vi "PC_Shot_Power.vi"(5 "Bounce T/F?":bool, 7 "Puck Selection":enum32{"PTFE", "Nylon"}(radio), 8 "Error In":errorcluster, 11 "PC Data":T1) -> (0 "Error Out":errorcluster, 2 "Kicker angle":dbl, 3 "Power %":dbl)   [LabVIEW 2017]
uses:
  pc_data.ctl
  <vilib>/vision/Image Controls.llb/IMAQ Image.ctl
  <vilib>/Utility/file.llb/Read Delimited Spreadsheet (DBL).vi
panel:
  in  "FF Bounce":dbl=0.66
  in  "FF Straight":dbl=1.68 format="%#_13g"
  out "Goal Y Bounce":dbl
  in  "Kicker Res":dbl=0.5
  out "Goal Y Straight":dbl
  in  "Friction PTFE":dbl=0.4
  in  "Puck Mass PTFE":dbl=0.0069
  in  "Friction Nylon":dbl=0.31
  in  "Puck Mass Nylon":dbl=0.0037
  out "Wall X Bounce":dbl
  out "Pot Position":dbl
  in  "Pendulum length":dbl=0.069
  in  "Pendulum mass":dbl=0.096
  out "Required E":dbl
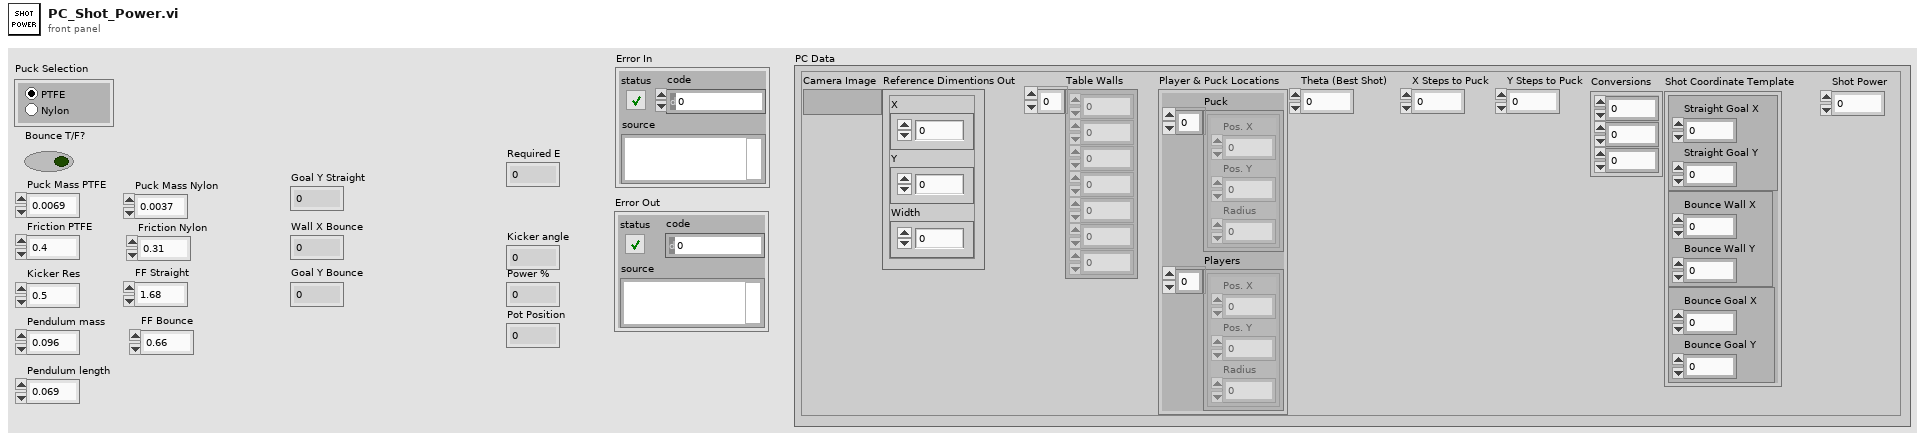
[diagram p1: front panel]
types:
  T1 = typedef "pc_data.ctl" = cluster{"Camera Image":T2, "Reference Dimentions Out":cluster{"X":dbl, "Y":dbl, "Width":dbl}, "Table Walls":sgl[], "Player & Puck Locations":cluster{"Puck":cluster{"Pos. X":i32, "Pos. Y":i32, "Radius":i32}[], "Players":cluster{"Pos. X":i32, "Pos. Y":i32, "Radius":i32}[]}, "Theta (Best Shot)":dbl, "X Steps to Puck":dbl, "Y Steps to Puck":dbl, "Conversions":cluster{dbl, dbl, dbl}, "Shot Coordinate Template":cluster{cluster{"Straight Goal X":sgl, "Straight Goal Y":dbl}, cluster{"Bounce Wall X":dbl, "Bounce Wall Y":sgl}, cluster{"Bounce Goal X":sgl, "Bounce Goal Y":dbl}}, "Shot Power":dbl}
  T2 = typedef "IMAQ Image.ctl" = refnum<image>
  T3 = cluster{"Pos. X":i32, "Pos. Y":i32, "Radius":i32}[]
  T4 = cluster{cluster{"Straight Goal X":sgl, "Straight Goal Y":dbl}, cluster{"Bounce Wall X":dbl, "Bounce Wall Y":sgl}, cluster{"Bounce Goal X":sgl, "Bounce Goal Y":dbl}}
  T5 = cluster{"Straight Goal X":sgl, "Straight Goal Y":dbl}
  T6 = cluster{"Bounce Wall X":dbl, "Bounce Wall Y":sgl}
  T7 = cluster{"Bounce Goal X":sgl, "Bounce Goal Y":dbl}
  T8 = cluster{"Pos. X":i32, "Pos. Y":i32, "Radius":i32}
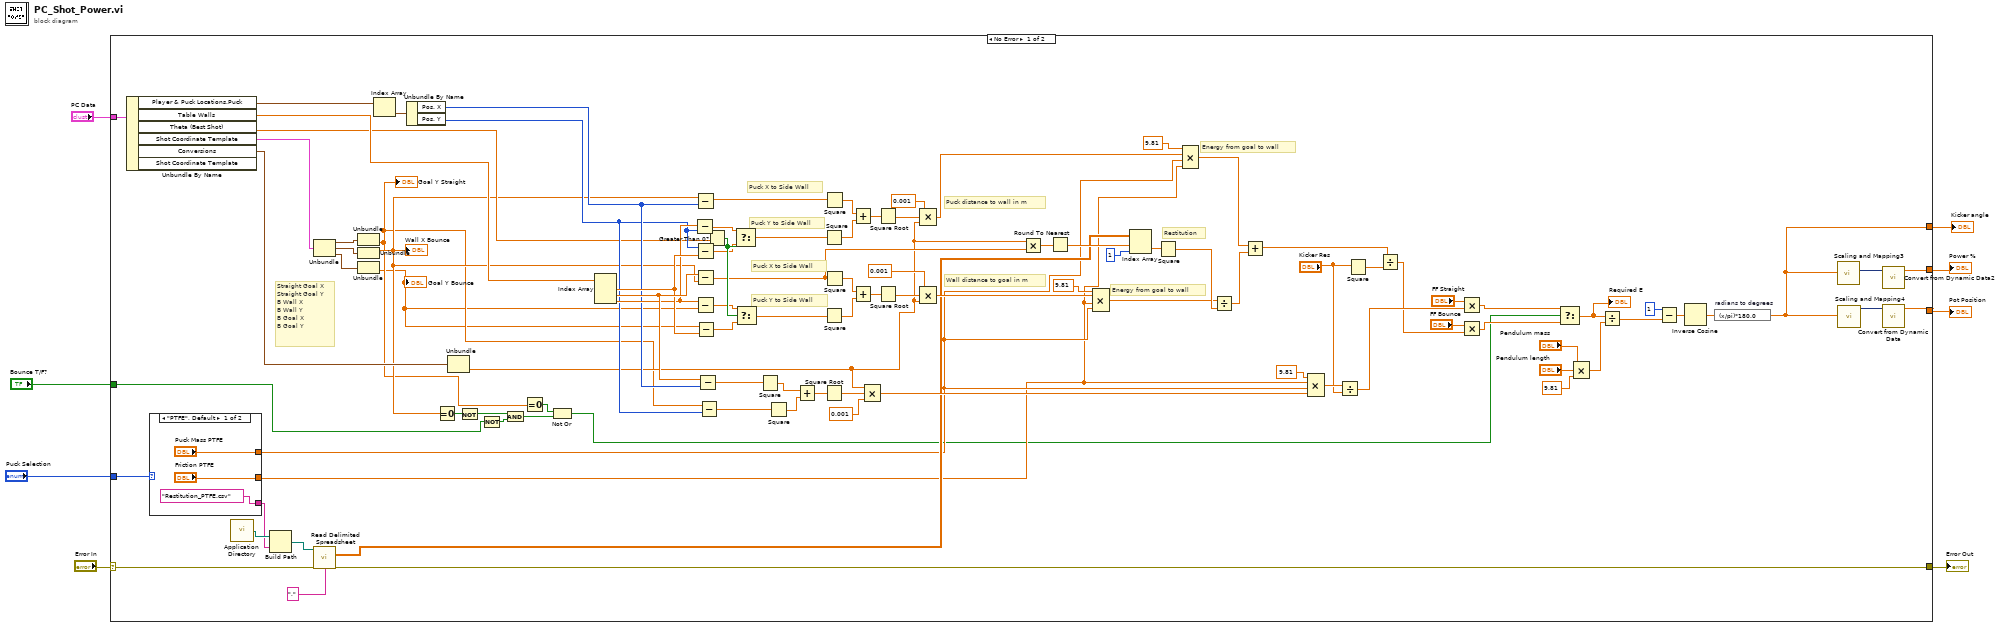
[diagram p0: block diagram]
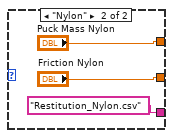
[diagram p2: hidden frame]
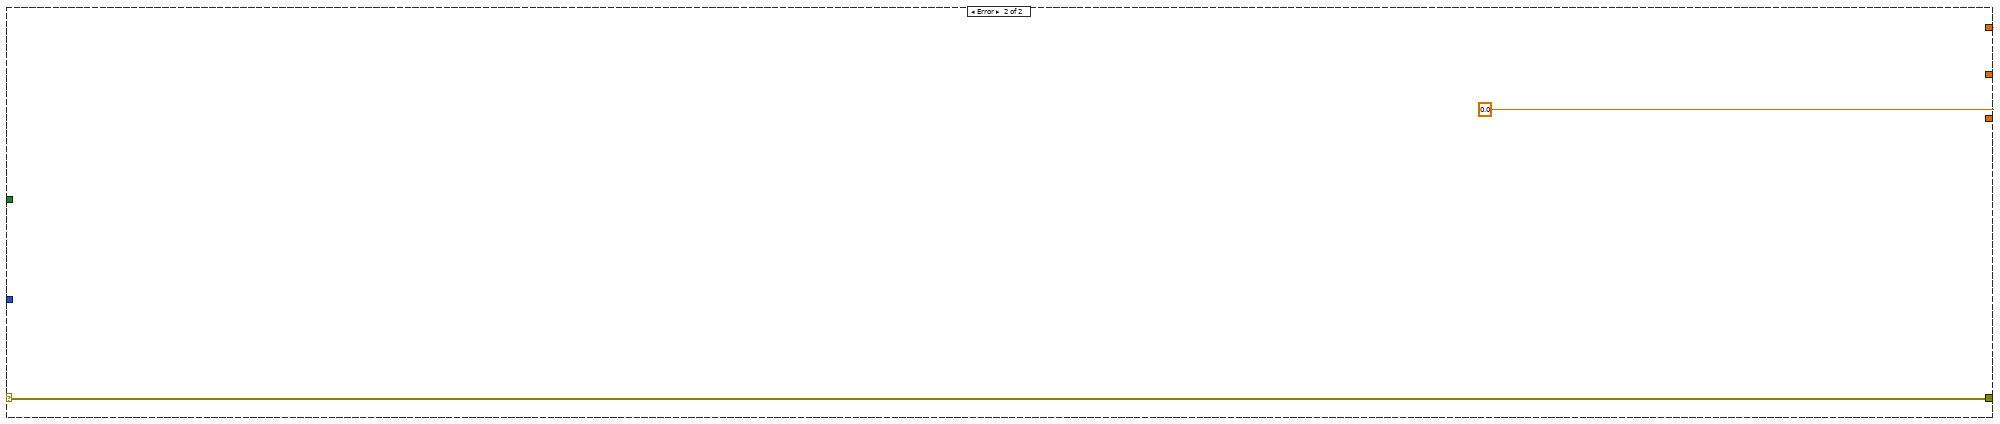
[diagram p3: hidden frame]
diagram:
  n1 = case shown="No Error" "Error In" {
    selector: "Error In" -> [w107 w116]
    tunnel: [w106 w116] -> w7
    tunnel: "Puck Selection" -> [w105 _]
    tunnel: "PC Data" -> [w102 _]
    tunnel: [w24 0.0] -> w4
    tunnel: [w25 _] -> w3
    tunnel: [w22 _] -> w2
    tunnel: "Bounce T/F?" -> [w13 _]
    frame No Error {
      # "Energy from goal to wall"
      # "Restitution"
      # "Energy from goal to wall"
      # "Puck X to Side Wall"
      # "Puck Y to Side Wall"
      # "Wall distance to goal in m"
      # "Puck distance to wall in m"
      # "Puck Y to Side Wall"
      # "Puck X to Side Wall"
      # "Straight Goal X\nStraight Goal Y\nB Wall X\nB Wall Y\nB Goal X\nB Goal Y"
      n2 = Unbundle By Name(w102) -> ("Player & Puck Locations.Puck"=w104:T3, "Table Walls"=w37:sgl[], "Theta (Best Shot)"=w34:dbl, "Shot Coordinate Template"=w98:T4, "Conversions"=w94:cluster{dbl, dbl, dbl})  [unwired: 1 out]
      n3 = case shown="\"PTFE\", Default" w105 {
        tunnel: ["Puck Mass PTFE" "Puck Mass Nylon"] -> w31
        tunnel: ["Friction PTFE" "Friction Nylon"] -> w30
        tunnel: ["Restitution_PTFE.csv" "Restitution_Nylon.csv"] -> w99
        frame "PTFE", Default {
        }
        frame "Nylon" {
        }
      }
      n4 = call <vilib>:"Application Directory.vi"() -> ("Application Directory"=w100:path)
      n5 = Build Path(base path=w100, name or relative path=w99) -> (appended path=w101:path)
      n6 = Unbundle(w98) -> (w97:T5, w96:T6, w95:T7)
      n7 = call-poly <vilib>:"Read Delimited Spreadsheet.vi"("file path (dialog if empty)"=w101, "error in (no error)"=w107, "delimiter (\\t)"="," ("delimiter (\\t)")) -> ("all rows"=w32:dbl[][], "error out"=w106:errorcluster)  [unwired: 7 in, 4 out]
      n8 = Unbundle(w97) -> ("Straight Goal Y"=w10:dbl)  [unwired: 1 out]
      "Goal Y Straight" <- w10
      n9 = Unbundle(w96) -> ("Bounce Wall X"=w11:dbl)  [unwired: 1 out]
      "Wall X Bounce" <- w11
      n10 = Unbundle(w95) -> ("Bounce Goal Y"=w9:dbl)  [unwired: 1 out]
      "Goal Y Bounce" <- w9
      n11 = Index Array(array=w104) -> (element=w103:T8)  [unwired: 1 in]
      n12 = Unbundle By Name(w103) -> ("Pos. X"=w36:i32, "Pos. Y"=w35:i32)
      n13 = Equal To 0?(x=w11) -> (x = 0?=w17:bool)
      n14 = Unbundle(w94) -> (w33:dbl)  [unwired: 2 out]
      n15 = Not(x=w17) -> (.not. x?=w16:bool)
      n16 = Not(x=w13) -> (.not. x?=w15:bool)
      n17 = And(x=w16, y=w15) -> (x .and. y?=w18:bool)
      n18 = Equal To 0?(x=w10) -> (x = 0?=w12:bool)
      n19 = Not Or(1:w18, 2:w12) -> (0:w14:bool)
      n20 = Index Array(array=w37) -> (element #1=w62:sgl, element #2=w84:sgl, element #3=w61:sgl)  [unwired: 3 in]
      n21 = Subtract(x=w61, y=w35) -> (x-y=w47:sgl)
      n22 = Subtract(x=w11, y=w36) -> (x-y=w50:dbl)
      n23 = Subtract(x=w35, y=w62) -> (x-y=w48:sgl)
      n24 = Subtract(x=w84, y=w11) -> (x-y=w65:dbl)
      n25 = Subtract(x=w61, y=w9) -> (x-y=w60:dbl)
      n26 = Subtract(x=w9, y=w62) -> (x-y=w59:dbl)
      n27 = Subtract(x=w84, y=w36) -> (x-y=w81:sgl)
      n28 = Subtract(x=w10, y=w35) -> (x-y=w80:dbl)
      n29 = Greater Than 0?(x=w34) -> (x > 0?=w85:bool)
      n30 = Select(t=w47, s=w85, f=w48) -> (s? t:f=w49:sgl)
      n31 = Select(t=w60, s=w85, f=w59) -> (s? t:f=w63:dbl)
      n32 = Square(x=w81) -> (x^2=w78:sgl)
      n33 = Square(x=w80) -> (x^2=w79:dbl)
      n34 = Add(x=w78, y=w79) -> (x+y=w77:dbl)
      n35 = Square(x=w49) -> (x^2=w52:sgl)
      n36 = Square(x=w63) -> (x^2=w57:dbl)
      n37 = Square Root(x=w77) -> (sqrt(x)=w76:dbl)
      n38 = Square(x=w50) -> (x^2=w51:dbl)
      n39 = Square(x=w65) -> (x^2=w58:dbl)
      n40 = Add(x=w51, y=w52) -> (x+y=w53:dbl)
      n41 = Add(x=w58, y=w57) -> (x+y=w56:dbl)
      n42 = Compound Arithmetic op=MULTIPLY(w33, w76, 0.001 ("value")) -> (w82:dbl)
      n43 = Square Root(x=w53) -> (sqrt(x)=w54:dbl)
      n44 = Square Root(x=w56) -> (sqrt(x)=w55:dbl)
      n45 = Compound Arithmetic op=MULTIPLY(0.001 ("value"), w54, w33) -> (w70:dbl)
      n46 = Compound Arithmetic op=MULTIPLY(0.001 ("value"), w55, w33) -> (w64:dbl)
      n47 = Multiply(x=w33, y=w65) -> (x*y=w66:dbl)
      n48 = Round To Nearest(number=w66) -> (nearest integer value=w67:dbl)
      n49 = Compound Arithmetic op=MULTIPLY(9.81 ("value"), w64, w30, w31) -> (w69:dbl)
      n50 = Index Array(array=w32, index (row)=w67, index (col)=1 ("disabled index (col)")) -> (element=w68:dbl)
      n51 = Square(x=w68) -> (x^2=w73:dbl)
      n52 = Compound Arithmetic op=MULTIPLY(9.81 ("value"), w70, w31, w30) -> (w72:dbl)
      n53 = Divide(x=w69, y=w73) -> (x/y=w71:dbl)
      n54 = Add(x=w72, y=w71) -> (x+y=w75:dbl)
      n55 = Compound Arithmetic op=MULTIPLY(9.81 ("value"), w30, w31, w82) -> (w83:dbl)
      n56 = Divide(x=w83, y="Kicker Res") -> (x/y=w90:dbl)
      n57 = Square(x="Kicker Res") -> (x^2=w74:dbl)
      n58 = Divide(x=w75, y=w74) -> (x/y=w21:dbl)
      n59 = Multiply(x="FF Straight", y=w90) -> (x*y=w92:dbl)
      n60 = Multiply(x="FF Bounce", y=w21) -> (x*y=w20:dbl)
      n61 = Select(t=w92, s=w14, f=w20) -> (s? t:f=w29:dbl)
      "Required E" <- w29
      n62 = Compound Arithmetic op=MULTIPLY("Pendulum mass", "Pendulum length", 9.81) -> (w89:dbl)
      n63 = Divide(x=w29, y=w89) -> (x/y=w88:dbl)
      n64 = Subtract(x=1, y=w88) -> (x-y=w87:dbl)
      n65 = Inverse Cosine(1:w87) -> (0:w86:dbl)
      n66 = expression code="(x/pi)*180.0" "radians to degrees"(w86) -> (w24:dbl)
      n67 = call "Scaling and Mapping3"("Signals"=w24) -> ("Scaled Signals"=w91:dynamicdata)  [unwired: 9 in, 1 out]
      n68 = call "Scaling and Mapping4"("Signals"=w24) -> ("Scaled Signals"=w23:dynamicdata)  [unwired: 9 in, 1 out]
      n69 = call "Convert from Dynamic Data2"("Dynamic Data Type"=w91) -> ("Scalar"=w25:dbl)  [unwired: 3 in]
      n70 = call "Convert from Dynamic Data"("Dynamic Data Type"=w23) -> ("Scalar"=w22:dbl)  [unwired: 3 in]
    }
    frame Error {
    }
  }
  "Error Out" <- w7
  "Kicker angle" <- w4
  "Pot Position" <- w2
  "Power %" <- w3
